vi "ImPro - Reset Settings.vi"(8 "error in (no error)":errorcluster, 10 "UI Refs":T1, 11 "Boolean in":refnum<vi>) -> (0 "error out":errorcluster)   [LabVIEW 2023]
uses:
  Controls/ImPro - UI Refs.ctl
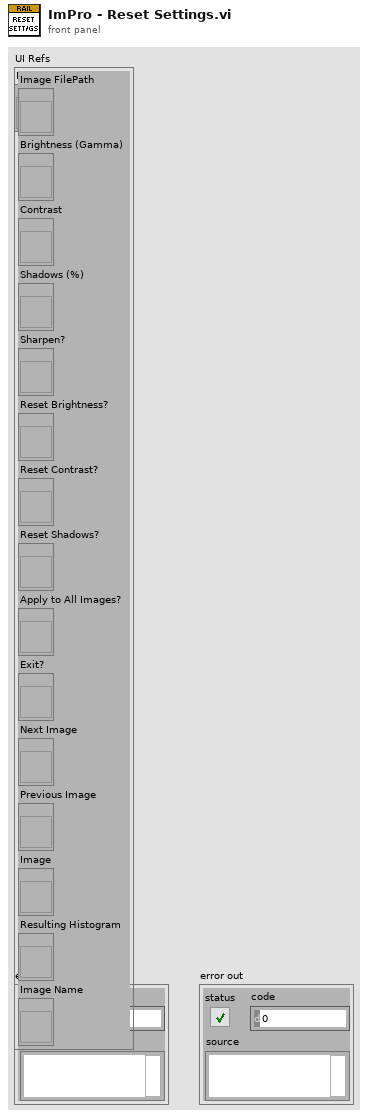
[diagram p1: front panel]
types:
  T1 = typedef "ImPro - UI Refs.ctl" = cluster{"Image FilePath":refnum<vi>, "Brightness (Gamma)":refnum<vi>, "Contrast":refnum<vi>, "Shadows (%)":refnum<vi>, "Sharpen?":refnum<vi>, "Reset Brightness?":refnum<vi>, "Reset Contrast?":refnum<vi>, "Reset Shadows?":refnum<vi>, "Apply to All Images?":refnum<vi>, "Exit?":refnum<vi>, "Next Image":refnum<vi>, "Previous Image":refnum<vi>, "Image":refnum<vi>, "Resulting Histogram":refnum<vi>, "Image Name":refnum<vi>}
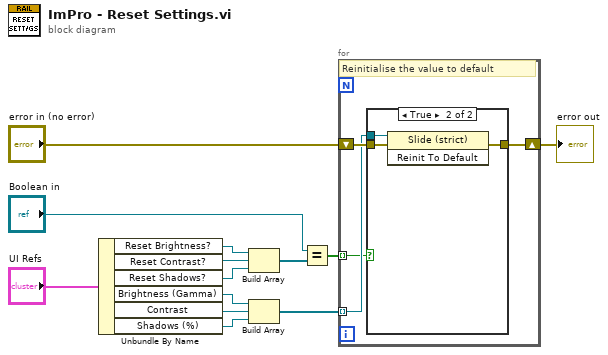
[diagram p0: block diagram]
diagram:
  n1 = Unbundle By Name("UI Refs") -> ("Reset Brightness?"=w2:refnum<vi>, "Reset Contrast?"=w3:refnum<vi>, "Reset Shadows?"=w6:refnum<vi>, "Brightness (Gamma)"=w7:refnum<vi>, "Contrast"=w8:refnum<vi>, "Shadows (%)"=w9:refnum<vi>)
  n2 = Build Array(w2, w3, w6) -> (w4:refnum<vi>[])
  n3 = Build Array(w7, w8, w9) -> (w10:refnum<vi>[])
  n4 = Equal?(x="Boolean in", y=w4) -> (x = y?=w11:bool[])
  n5 = for {
    tunnel: w10 -> [w15] mode=indexing
    tunnel: w11 -> [w14] mode=indexing
    shift-right: [w16] -> w13
    shift-left: "error in (no error)" -> [w17]
    # "Reinitialise the value to default"
    n6 = case shown="True" w14 {
      tunnel: w17 -> [w18 w21]
      tunnel: [w18 w20] -> w16
      tunnel: w15 -> [_ w19]
      frame False {
      }
      frame True {
        n7 = invoke class="Slide (strict)" method="Reinit To Default"(reference=w19, error in=w21) -> (error out=w20:errorcluster)  [unwired: 1 in, 2 out]
      }
    }
  }
  "error out" <- w13
